vi "Enable Menus.vi"(8 "error in (no error)":errorcluster, 10 "Valid":bool, 11 "Menu references":refnum<vi>[](array[refnum])) -> (0 "error out":errorcluster)   [LabVIEW 2019]
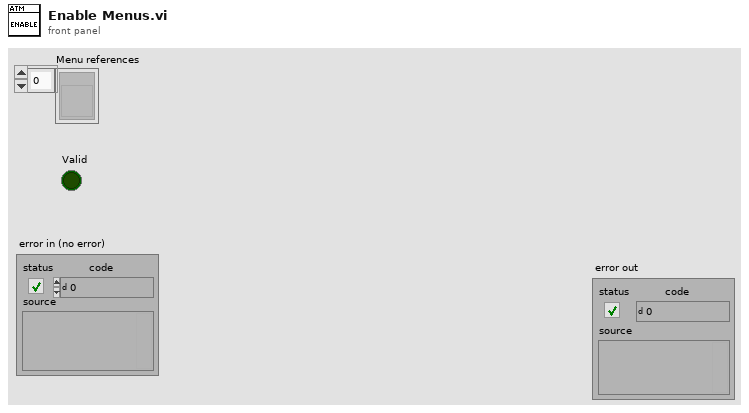
[diagram p1: front panel]
types:
  T1 = enum8{"Enabled", "Disabled", "Disabled and Grayed Out"}
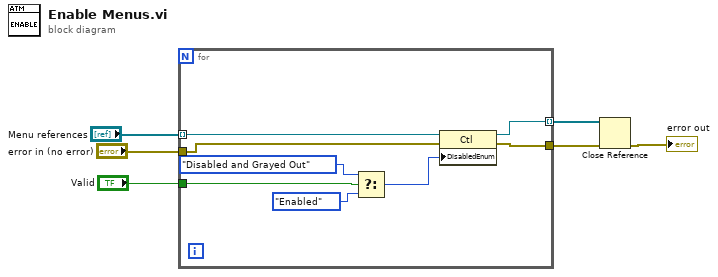
[diagram p0: block diagram]
diagram:
  n1 = for {
    tunnel: "Menu references" -> [w14] mode=indexing
    tunnel: "Valid" -> [w13]
    tunnel: "error in (no error)" -> [w9]
    tunnel: [w8] -> w4
    tunnel: [w7] -> w3 mode=indexing
    n2 = Select(t=T1."Disabled and Grayed Out" ("Disabled"), s=w13, f=T1."Enabled" ("Disabled")) -> (s? t:f=w10:T1)
    n3 = property class="Ctl"(reference=w14, error in=w9, "DisabledEnum"=w10) -> (reference out=w7:refnum<vi>, error out=w8:errorcluster)
  }
  n4 = Close Reference(reference=w3, error in (no error)=w4) -> (error out=→"error out":errorcluster)
